vi "Actor Core.vi"(8 "error in":errorcluster, 11 "Tracer-V in":refnum<class "Tracer-V.lvclass">) -> (0 "error out":errorcluster, 3 "Actor out":refnum<class "Actor.lvclass">)   [LabVIEW 2013, in "Tracer-V.lvclass"]
doc: "(<B>Filename</B>: Actor Framework.lvlib:Actor.lvclass:Actor Core.vi)\n\nReceives messages to the actor, reacts to them, and initiates any error handling that may shut the actor down.\n\nDescendant classes may override this VI to append parallel tasks for the actor to complete while it handles messages. Overrides use the Call Parent Method node."
uses:
  Tracer-V.lvclass
  <vilib>/ActorFramework/Actor/Actor.lvclass
  Logical Systems/Tracer/Tracer.lvclass
  Tracer-V.lvclass/Tracer-V.ctl
panel:
  out "Data":string
  out "Mouse Enter":string
  out "Traces":string[][](table)
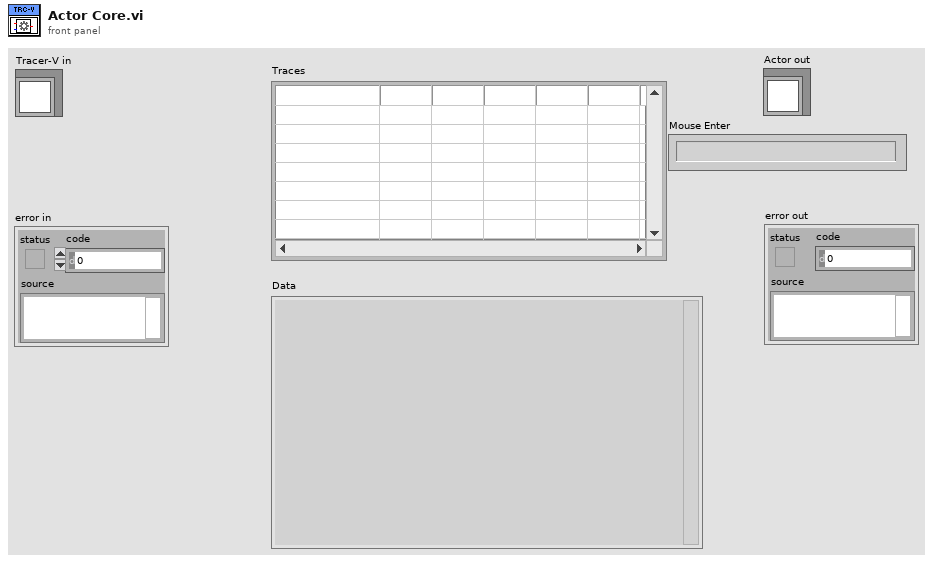
[diagram p1: front panel]
types:
  T1 = typedef "LVRowAndColumnTypeDef.ctl" = cluster{"Row":i32, "Column":i32}
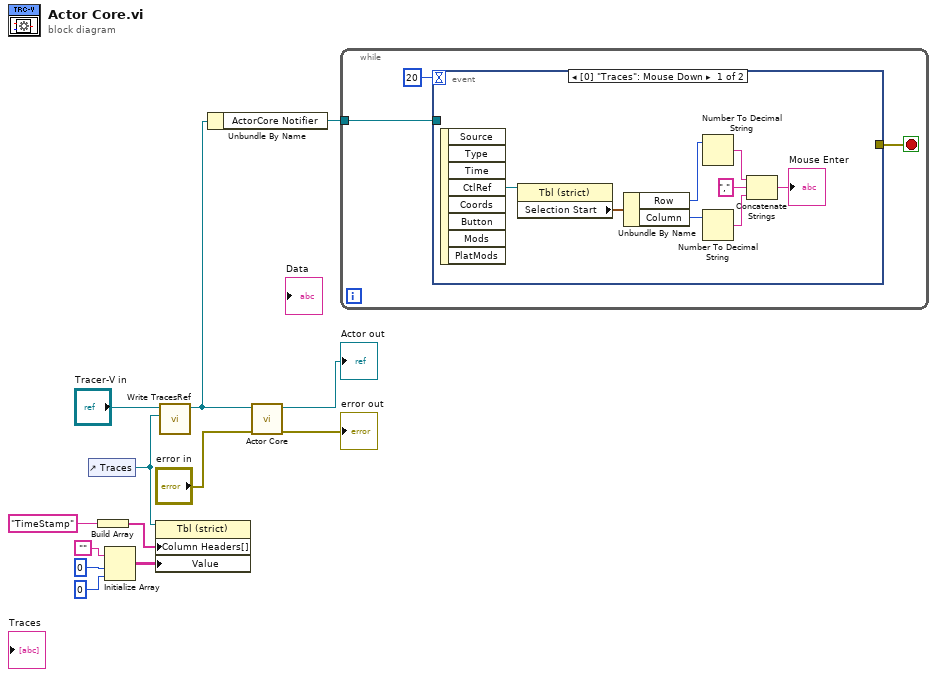
[diagram p0: block diagram]
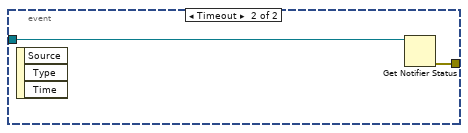
[diagram p2: hidden frame]
diagram:
  n1 = control-ref of="Traces"() -> (w10:refnum<vi>)
  n2 = Build Array("TimeStamp") -> (w8:string[])
  n3 = Initialize Array("", 0 ("dimension size"), 0 ("dimension size")) -> (w7:string[][])
  n4 = property class="Tbl (strict)"(reference=w10, "Column Headers[]"=w8, "Value"=w7) -> ()  [unwired: 1 in, 2 out]
  n5 = call-dynamic "Write TracesRef.vi"("TracesRef"=w10, "Tracer-V in"="Tracer-V in") -> ("Tracer-V out"=w2:refnum<class "Tracer-V.lvclass">)  [unwired: 8 in, 1 out]
  n6 = Unbundle By Name(w2) -> ("ActorCore Notifier"=w1:refnum<notifier>)
  n7 = call-parent "Actor Core.vi"("error in"="error in", "Actor in"=w2) -> ("error out"=→"error out":errorcluster, "Actor out"=→"Actor out":refnum<class "Actor.lvclass">)  [unwired: 8 in]
  n8 = while {
    tunnel: w1 -> [w16]
    stop <- w14 stop-if-true
    n9 = event shown="[0] \"Traces\": Mouse Down" {
      selector: _ -> [_ _]
      dyn-events: _ -> [_ _]
      timeout: 20 -> [_ _]
      tunnel: w16 -> [_ w26]
      tunnel: [_ w25] -> w14
      event "Traces": Mouse Down {
        n10 = event-data() -> ("CtlRef"=w24:refnum<vi>)  [unwired: 1 in, 7 out]
        n11 = property class="Tbl (strict)"(reference=w24) -> ("Selection Start"=w23:T1)  [unwired: 1 in, 2 out]
        n12 = Unbundle By Name(w23) -> ("Row"=w22:i32, "Column"=w21:i32)
        n13 = Number To Decimal String(number=w22) -> (decimal integer string=w20:string)  [unwired: 1 in]
        n14 = Number To Decimal String(number=w21) -> (decimal integer string=w18:string)  [unwired: 1 in]
        n15 = Concatenate Strings(w20, "," ("string"), w18) -> (→"Mouse Enter":string)
      }
      event Timeout {
        n16 = event-data() -> ()  [unwired: 1 in, 3 out]
        n17 = Get Notifier Status(notifier=w26) -> (error out=w25:errorcluster)  [unwired: 1 in, 4 out]
      }
    }
  }
